vi "_readUnicode.vi"(8 "error in (no error)":errorcluster, 11 "tJSONParser in":refnum<class "tJSONParser.lvclass">) -> (0 "error out":errorcluster, 2 "String Out":string, 3 "tJSONParser out":refnum<class "tJSONParser.lvclass">)   [LabVIEW 2013, in "JSON.lvlib" / "tJSONParser.lvclass"]
doc: "Reads in a unicode escape sequence of the form \\uxxxx, where x is a hexadecimal digit. If the xxxx is a control code, an error will be returned."
uses:
  tJSONParser.lvclass
  tJSONParser.lvclass/tJSONParser.ctl
  _error.ctl
  <vilib>/regexp/Match Regular Expression.xnode
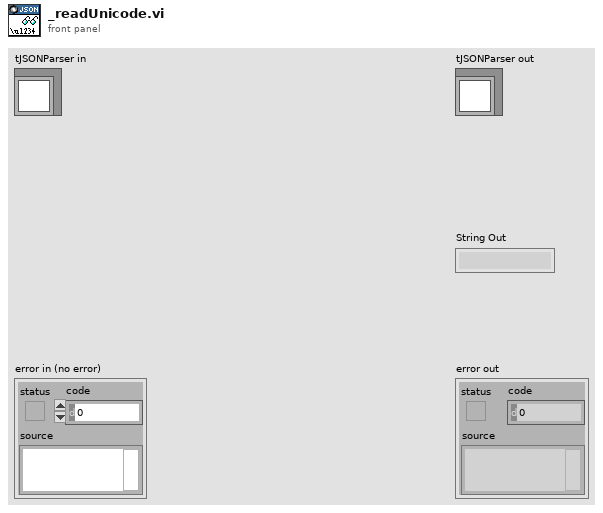
[diagram p1: front panel]
types:
  T1 = typedef "JSON.lvlib/tJSONParser.lvclass/_error.ctl" = enum16{"Missing Object Open", "Missing Pair Separator", "Missing Object End Or Separator", "Missing Pair String", "Unexpected Token", "Missing Array End Or Separator", "Invalid Escape Sequence", "Unexpected End Of File", "Invalid Unicode", "Unexpected End Of Line", "Invalid Numerical Constant"}
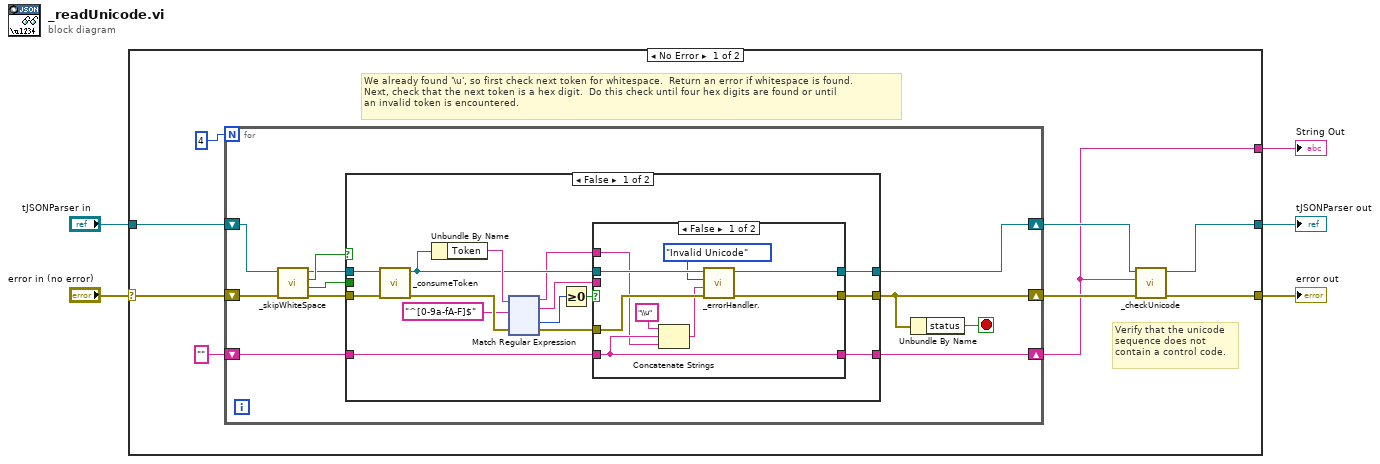
[diagram p0: block diagram]
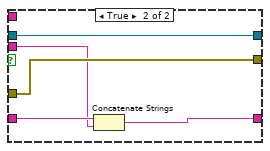
[diagram p2: hidden frame]
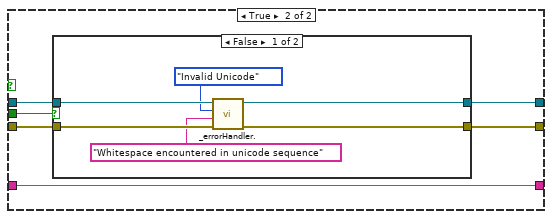
[diagram p3: hidden frame]
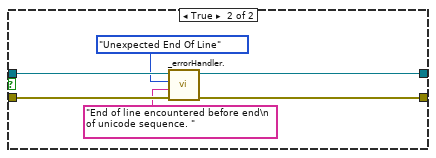
[diagram p4: hidden frame]
diagram:
  n1 = case shown="No Error" "error in (no error)" {
    selector: "error in (no error)" -> [w13 w184]
    tunnel: [w9 w184] -> w4
    tunnel: [w7 w185] -> w2
    tunnel: "tJSONParser in" -> [w12 w185]
    tunnel: [w6 _] -> w1
    frame No Error {
      # "Verify that the unicode\nsequence does not\ncontain a control code."
      # "We already found '\\u', so first check next token for whitespace.  Return an error if whitespace is found.\nNext, check that the next token is a hex digit.  Do this check until four hex digits are found or until \nan invalid token is encountered."
      n2 = for {
        N: 4 ("Numeric") -> [_]
        shift-right: [w18] -> w10
        shift-left: w13 -> [w25]
        shift-right: [w19] -> w8
        shift-left: w12 -> [w24]
        shift-right: [w15] -> w6
        shift-left: "" -> [w16]
        stop <- w17 stop-if-true
        n3 = call "_skipWhiteSpace.vi"("error in (no error)"=w25, "JSON Parser In"=w24) -> ("error out"=w23:errorcluster, "EOL Found?"=w21:bool, "White Space Found?"=w22:bool, "JSON Parser Out"=w20:refnum<class "tJSONParser.lvclass">)  [unwired: 5 in, 1 out]
        n4 = case shown="False" w22 {
          tunnel: w23 -> [w40 w171]
          tunnel: [w32 w170] -> w18
          tunnel: w21 -> [_ w169]
          tunnel: w20 -> [w39 w168]
          tunnel: [w31 w167] -> w19
          tunnel: w16 -> [w28 w166]
          tunnel: [w27 w166] -> w15
          frame False {
            n5 = call "_consumeToken.vi"("error in (no error)"=w40, "JSON Parser In"=w39) -> ("error out"=w38:errorcluster, "JSON Parser Out"=w30:refnum<class "tJSONParser.lvclass">)  [unwired: 8 in]
            n6 = Unbundle By Name(w30) -> ("Token"=w37:string)
            n7 = xnode "Match Regular Expression"("input string"=w37, "regular expression"="^[0-9a-fA-F]$", "error in"=w38) -> ("before match"=w26:string, "whole match"=w29:string, "offset past match"=w35:i32, "error out"=w33:errorcluster)  [unwired: 3 in, 1 out]
            n8 = Greater Or Equal To 0?(x=w35) -> (x >= 0?=w34:bool)
            n9 = case shown="False" w34 {
              tunnel: w33 -> [w49 w54]
              tunnel: [w48 w54] -> w32
              tunnel: [w47 w53] -> w31
              tunnel: w30 -> [w46 w53]
              tunnel: w29 -> [_ w51]
              tunnel: w28 -> [w42 w52]
              tunnel: [w42 w50] -> w27
              tunnel: w26 -> [w41 _]
              frame False {
                n10 = Concatenate Strings("\\u" ("string"), w42, w41) -> (w44:string)
                n11 = call "_errorHandler..vi"("error in (no error)"=w49, "Additional Text"=w44, "Error Type"=_error."Invalid Unicode", "JSON Parser In"=w46) -> ("error out"=w48:errorcluster, "JSON Parser Out"=w47:refnum<class "tJSONParser.lvclass">)  [unwired: 6 in]
              }
              frame True {
                n12 = Concatenate Strings(w52, w51) -> (w50:string)
              }
            }
          }
          frame True {
            n13 = case shown="False" w169 {
              tunnel: w171 -> [w177 w183]
              tunnel: [w176 w182] -> w170
              tunnel: w168 -> [w175 w181]
              tunnel: [w174 w180] -> w167
              frame False {
                n14 = call "_errorHandler..vi"("error in (no error)"=w177, "Additional Text"="Whitespace encountered in unicode sequence", "Error Type"=_error."Invalid Unicode", "JSON Parser In"=w175) -> ("error out"=w176:errorcluster, "JSON Parser Out"=w174:refnum<class "tJSONParser.lvclass">)  [unwired: 6 in]
              }
              frame True {
                n15 = call "_errorHandler..vi"("error in (no error)"=w183, "Additional Text"="End of line encountered before end\n of unicode sequence. ", "Error Type"=_error."Unexpected End Of Line", "JSON Parser In"=w181) -> ("error out"=w182:errorcluster, "JSON Parser Out"=w180:refnum<class "tJSONParser.lvclass">)  [unwired: 6 in]
              }
            }
          }
        }
        n16 = Unbundle By Name(w18) -> ("status"=w17:bool)
      }
      n17 = call "_checkUnicode.vi"("error in (no error)"=w10, "String In"=w6, "tJSONParser in"=w8) -> ("error out"=w9:errorcluster, "tJSONParser out"=w7:refnum<class "tJSONParser.lvclass">)  [unwired: 7 in]
    }
    frame Error {
    }
  }
  "error out" <- w4
  "tJSONParser out" <- w2
  "String Out" <- w1
